vi "writeFile.vi"(8 "error in (no error)":errorcluster caption="entrée d'erreur (pas d'erreur)", 10 "script":string, 11 "Python en entrée":refnum<class "Python.lvclass">) -> (0 "error out":errorcluster caption="sortie d'erreur", 3 "Python en sortie":refnum<class "Python.lvclass">)   [LabVIEW 2020, in "Python.lvclass"]
uses:
  Python.lvclass
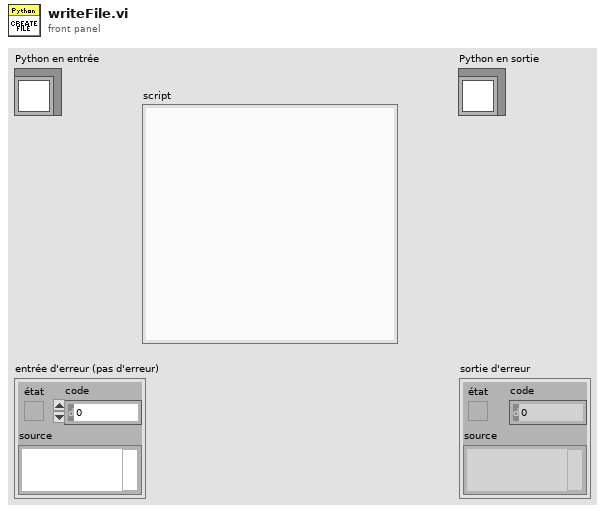
[diagram p1: front panel]
types:
  T1 = enum16{"open", "replace", "create", "open or create", "replace or create", "replace or create with confirmation"}
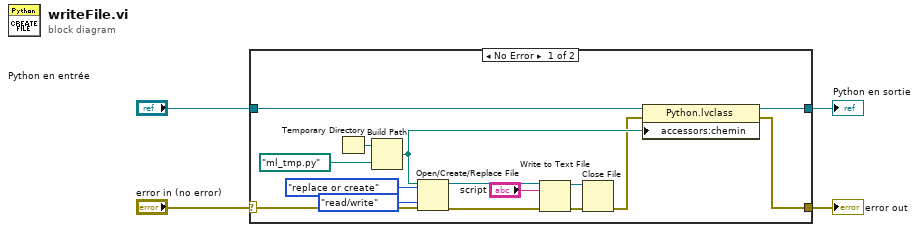
[diagram p0: block diagram]
diagram:
  n1 = case shown="No Error" "error in (no error)" {
    selector: "error in (no error)" -> [w17 w21]
    tunnel: [w11 w21] -> w3
    tunnel: [w6 w20] -> w1
    tunnel: "Python en entrée" -> [w9 w20]
    frame No Error {
      n2 = Temporary Directory() -> (w8:path)
      n3 = Build Path(base path=w8, name or relative path=path "ml_tmp.py" ("nom ou chemin relatif")) -> (appended path=w7:path)
      n4 = Open/Create/Replace File(file path (use dialog)=w7, error in=w17, operation (0:open)=T1."replace or create" ("opération (0 : open)"), access (0:read/write)=enum16{"read/write", "read-only", "write-only"}."read/write" ("accès (0 : read/write)")) -> (refnum out=w16:refnum<file>, error out=w14:errorcluster)  [unwired: 2 in, 1 out]
      n5 = Write to Text File(file (use dialog)=w16, text="script", error in=w14) -> (refnum out=w12:refnum<file>, error out=w13:errorcluster)  [unwired: 1 in, 1 out]
      n6 = Close File(refnum=w12, error in=w13) -> (error out=w5:errorcluster)  [unwired: 1 out]
      n7 = property class="Python.lvclass"(reference=w9, error in=w5, "accessors:chemin"=w7) -> (reference out=w6:refnum<class "Python.lvclass">, error out=w11:errorcluster)
    }
    frame Error {
    }
  }
  "error out" <- w3
  "Python en sortie" <- w1
